vi "Compressor With Cylinder.vi"() -> ()   [LabVIEW 2023]
doc: "Compressor with Cylinder \n\nThis example shows how to control a compressor, extend and retract a cylinder, and optionally use a limit switch to retract automatically.\n\nThis example works with the PCM (Pneumatic Control Module) communicating with the roboRIO over CAN bus. The PCM must also be supplied with 12V DC from the PDP (Power Distribution Panel).\n\nThe Compressor, Pressure Switch, and Solenoids are all wired to the PCM \n\nThe Limit Switch is wired to DIO 9. It causes the cylinder to retract when the Auto Retract button is pressed.\n\nRefer to the Pneumatics Manual for air connections. Your pneumatics setup should include a compressor, pressure switch, tank, regulator, valve, flow controls, cylinder, plug valve, etc.\n\nTo run this example you should have a pneumatic system with air pressure connected to the P input on the SMC double solenoid valve. The A output of the valve should be connected via a flow control to the backend of a cylinder. The B output of the valve should be connected via a flow control to the frontend of a cylinder. When the cylinder is extended, it should physically depress the Limit Switch.\n\nWith the VI running, pressing the Extend button will push the cylinder shaft out, and pressing the Retract button will pull it back. Notice that the Extend and Retract buttons have their Mechanical Action set to Latch When Pressed. This means they stay pressed (ON) until they are read by the program, then they return to the OFF position. This works because once the SMC solenoid valve is pulled one direction, it stays in that position until it is pulled in the opposite direction - it only needs to be momentarily energized. The Auto Retract button can be used to make the cylinder return automatically. With the Auto Retract button ON, pressing the Extend button will push the cylinder out, and it will retract when it hits the limit switch.\n\nThis example expects a USB cable connected from your development PC to the Type B USB Jack (next to the power input) on the roboRIO.\n\nThis example expects the Driver Station to be running."
uses:
  <vilib>/Rock Robotics/WPI/Solenoid/WPI_SolenoidChannel.ctl
  <vilib>/Rock Robotics/WPI/Solenoid/WPI_SolenoidValue.ctl
  <vilib>/Rock Robotics/WPI/Solenoid/WPI_SolenoidOpenDouble.vi
  <vilib>/Rock Robotics/WPI/Solenoid/WPI_SolenoidSetEnum.vi
panel:
  in  "Back 2":bool
  in  "Fwd 2":bool
  in  "Extend Solenoid Channel 2":T1=enum."Solenoid 1"
  in  "Retract Solenoid Channel 2":T1
  in  "Select a PD device by clicking on the image below":u16(ring) items=["CTRE Pneumatic Module", "REV Pneumatics Hub"]
  out "Compressor Running":bool
  in  "Fwd 1":bool
  in  "Retract Solenoid Channel":T1
  in  "Extend Solenoid Channel":T1=enum."Solenoid 1"
  out "Compressor Monitoring":bool
  in  "stop":bool
  in  "Back 1":bool
  # "Set these inputs before running."
  # "roboRIO Wiring Diagram"
  # "when extended, the cylinder should depress this"
  # "Limit\nSwitch"
  # "These can be set while running."
  # "Output information."
  # "COM"
  # "NC"
  # "NO"
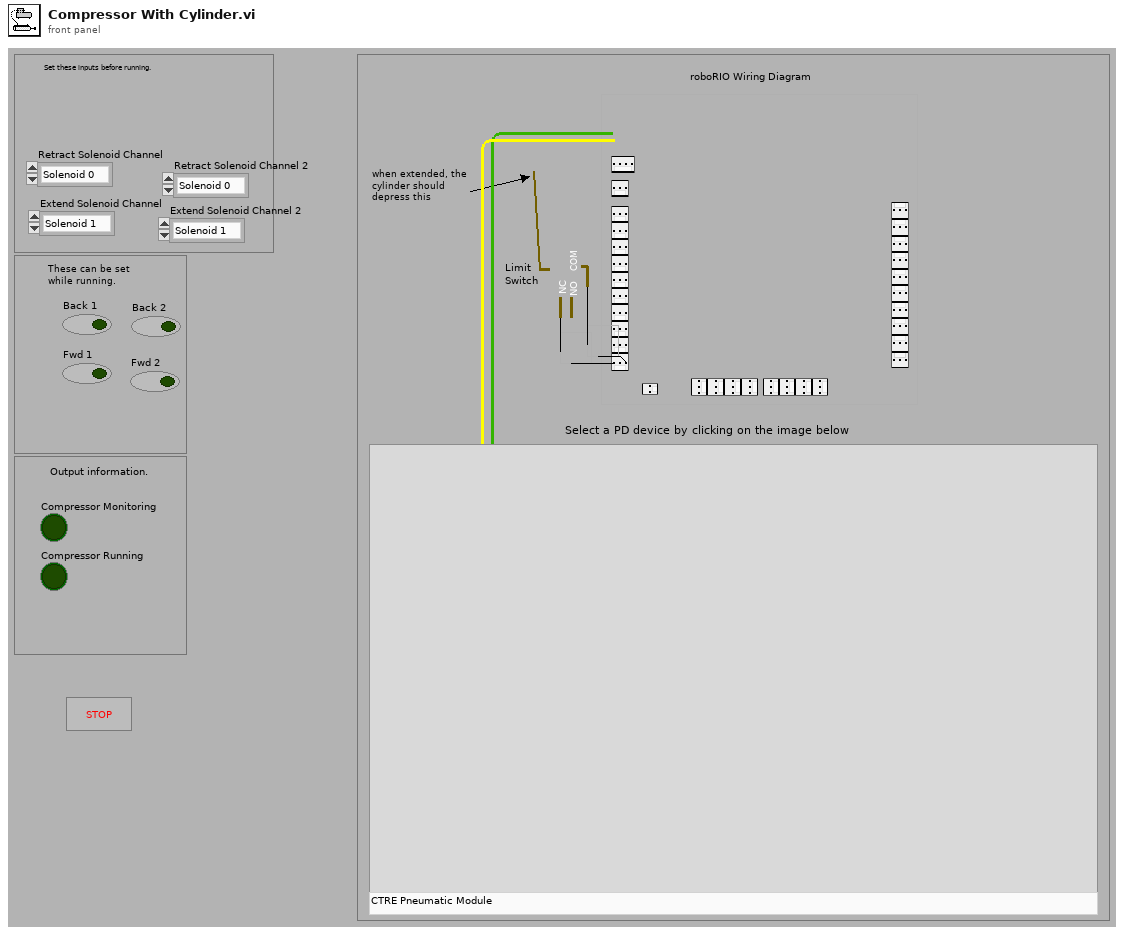
[diagram p1: front panel]
types:
  T1 = typedef "WPI_SolenoidChannel.ctl" = enum8{"Solenoid 0", "Solenoid 1", "Solenoid 2", "Solenoid 3", "Solenoid 4", "Solenoid 5", "Solenoid 6", "Solenoid 7", "Solenoid 8", "Solenoid 9", "Solenoid 10", "Solenoid 11", "Solenoid 12", "Solenoid 13", "Solenoid 14", "Solenoid 15", "Invalid"}
  T2 = typedef "WPI_CompressorDevRef.ctl" = cluster{"DevStatus":errorcluster, "Pneumatics Control Module":u8}
  T3 = typedef "WPI_SolenoidDevRef.ctl" = cluster{"DevStatus":errorcluster, "Pneumatics Control Module":u8, "Forward Solenoid Channel":T1, "Reverse Solenoid Channel":T1}
  T4 = typedef "WPI_SolenoidValue.ctl" = enum16{"Off", "On", "Forward", "Reverse"}
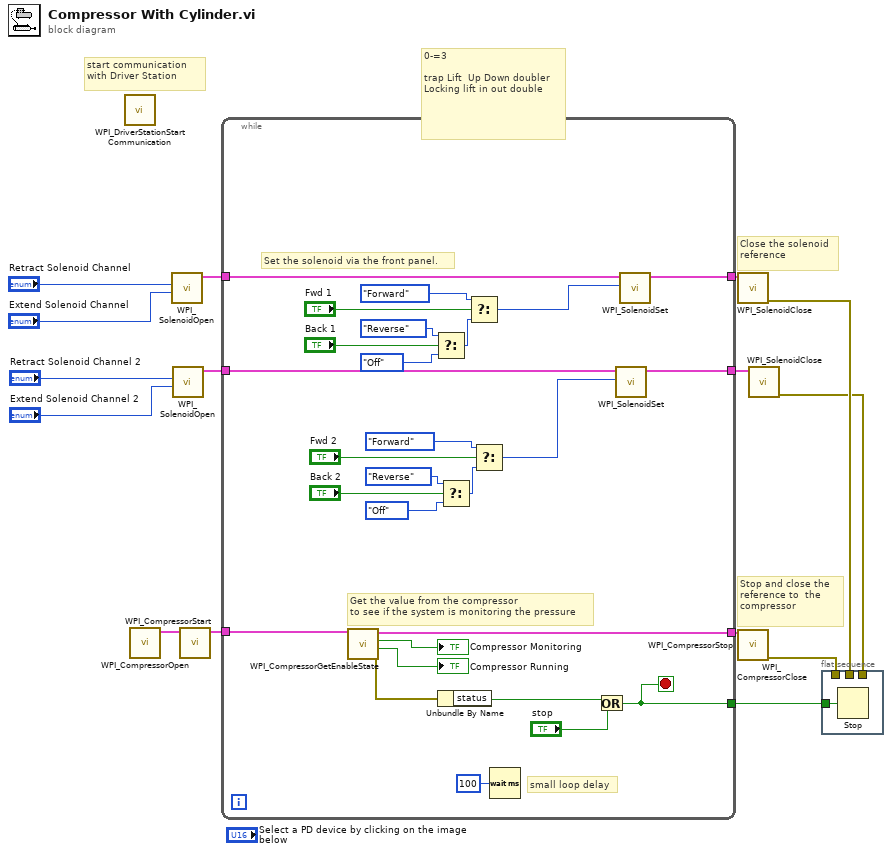
[diagram p0: block diagram]
diagram:
  # "0-=3\n\ntrap Lift  Up Down doubler\nLocking lift in out double"
  # "Close the solenoid\nreference"
  # "start communication with Driver Station"
  # "Stop and close the reference to  the compressor"
  n1 = call <vilib>:"WPI_DriverStationStart Communication.vi"() -> ()  [unwired: 3 in, 9 out]
  n2 = call <vilib>:"WPI_CompressorOpen.vi"() -> ("CompressorDevRef"=w9:T2)  [unwired: 14 in, 1 out]
  n3 = call-poly <vilib>:"WPI_SolenoidOpen.vi"("Reverse Solenoid Channel"="Extend Solenoid Channel", "Forward Solenoid Channel"="Retract Solenoid Channel") -> ("SolenoidDevRef"=w12:T3)  [unwired: 2 in, 7 out]
  n4 = call-poly <vilib>:"WPI_SolenoidOpen.vi"("Reverse Solenoid Channel"="Extend Solenoid Channel 2", "Forward Solenoid Channel"="Retract Solenoid Channel 2") -> ("SolenoidDevRef"=w3:T3)  [unwired: 2 in, 7 out]
  n5 = call <vilib>:"WPI_CompressorStart.vi"("CompressorDevRef"=w9) -> ("CompressorDevRef"=w15:T2)  [unwired: 2 in, 8 out]
  n6 = while {
    tunnel: w15 -> [w43]
    tunnel: [w42] -> w14
    tunnel: [w40] -> w8
    tunnel: w12 -> [w35]
    tunnel: [w27] -> w13
    tunnel: w3 -> [w19]
    tunnel: [w17] -> w2
    stop <- w40 stop-if-true
    # "small loop delay"
    # "Get the value from the compressor \nto see if the system is monitoring the pressure"
    # "Set the solenoid via the front panel."
    n7 = call <vilib>:"WPI_CompressorGetEnableState.vi"("CompressorDevRef"=w43) -> ("error out"=w38:errorcluster, "Compressor Running"=→"Compressor Running":bool, "Enabled"=→"Compressor Monitoring":bool, "CompressorDevRef"=w42:T2)  [unwired: 1 in, 6 out]
    n8 = Select(t=WPI_SolenoidValue."Reverse" ("Value"), s="Back 1", f=WPI_SolenoidValue."Off" ("Value")) -> (s? t:f=w29:T4)
    n9 = Unbundle By Name(w38) -> ("status"=w37:bool)
    n10 = Select(t=WPI_SolenoidValue."Reverse" ("Value"), s="Back 2", f=WPI_SolenoidValue."Off" ("Value")) -> (s? t:f=w24:T4)
    n11 = Select(t=WPI_SolenoidValue."Forward" ("Value"), s="Fwd 1", f=w29) -> (s? t:f=w26:T4)
    n12 = Select(t=WPI_SolenoidValue."Forward" ("Value"), s="Fwd 2", f=w24) -> (s? t:f=w18:T4)
    n13 = Wait (ms)(milliseconds to wait=u32 100) -> ()  [unwired: 1 out]
    n14 = Or(x=w37, y="stop") -> (x .or. y?=w40:bool)
    n15 = call-poly <vilib>:"WPI_SolenoidSet.vi"("Value"=w18, "SolenoidDevRef"=w19) -> ("SolenoidDevRef"=w17:T3)  [unwired: 1 in, 8 out]
    n16 = call-poly <vilib>:"WPI_SolenoidSet.vi"("Value"=w26, "SolenoidDevRef"=w35) -> ("SolenoidDevRef"=w27:T3)  [unwired: 1 in, 8 out]
  }
  n17 = call <vilib>:"WPI_SolenoidClose.vi"("SolenoidDevRef"=w13) -> ("error out"=w6:errorcluster)  [unwired: 1 in, 9 out]
  n18 = call <vilib>:"WPI_CompressorStop.vi"("CompressorDevRef"=w14) -> ("CompressorDevRef"=w16:T2)  [unwired: 1 in, 9 out]
  n19 = call <vilib>:"WPI_CompressorClose.vi"("CompressorDevRef"=w16) -> ("error out"=w7:errorcluster)  [unwired: 1 in, 9 out]
  n20 = call <vilib>:"WPI_SolenoidClose.vi"("SolenoidDevRef"=w2) -> ("error out"=w1:errorcluster)  [unwired: 1 in, 9 out]
  n21 = flat-sequence {
    tunnel: w8 -> [w44]
    tunnel: w7 -> [_]
    tunnel: w6 -> [_]
    tunnel: w1 -> [_]
    frame #0 {
      n22 = Stop(stop? (T)=w44) -> ()
    }
  }
